vi "Send Set-Point Driver Stop Message.vi"   [LabVIEW 2013]
uses:
  Set-Point Driver Messages.ctl
types:
  T1 = typedef "Set-Point Driver Messages.ctl" = enum16{"Begin Enforcement", "Cease Enforcement"}
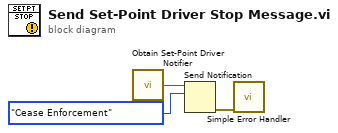
[diagram p0: block diagram]
diagram:
  n1 = call "Obtain Set-Point Driver Notifier.vi"() -> ("Set-Point Driver Notifier"=w3:refnum<notifier>)
  n2 = Send Notification(notification=Set-Point_Driver_Messages."Cease Enforcement", notifier=w3) -> (error out=w1:errorcluster)  [unwired: 1 in, 1 out]
  n3 = call <vilib>:"Simple Error Handler.vi"("error in (no error)"=w1) -> ()  [unwired: 4 in, 5 out]
